vi "Speed Control.vi"(6 "Multiple":dbl, 8 "Down":bool, 9 "Up":bool, 10 "Left Joystick":dbl, 11 "Right Joystick":dbl) -> (0 "Speed":dbl, 2 "Left Motor":dbl, 3 "Right Output":dbl)   [LabVIEW 2016]
doc: "This VI was created to demonstrate common functions used in Labview. It incriments/decrements a value based on the press of Up/Down by a value of multiple. The zero terminal sets the value to zero. The motor input in is multiplied by this value (-1<x<1) to control the maximum speed."
panel:
  in  "Zero":bool
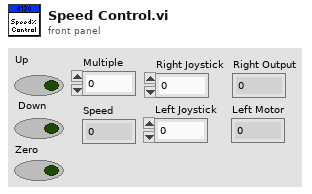
[diagram p1: front panel]
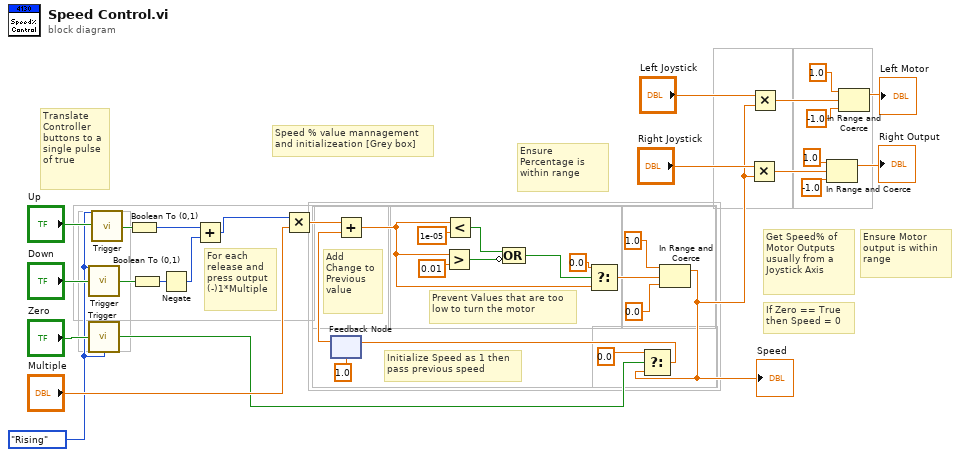
[diagram p0: block diagram]
diagram:
  w1 = enum16{"Falling", "Rising", "Both"}."Rising" ("Enum")
  # "Speed % value mannagement and initializeation [Grey box]"
  # "Get Speed% of Motor Outputs usually from a Joystick Axis"
  # "Ensure Motor output is within range"
  # "Initialize Speed as 1 then pass previous speed"
  # "If Zero == True then Speed = 0"
  # "Ensure Percentage is within range"
  # "Prevent Values that are too low to turn the motor"
  # "For each release and press output (-)1*Multiple"
  # "Translate Controller buttons to a single pulse of true"
  # "Add Change to Previous value"
  n1 = call "Trigger.vi"("Enum"=w1, "Button"="Down") -> ("Trigger"=w27:bool)  [unwired: 13 in]
  n2 = call "Trigger.vi"("Enum"=w1, "Button"="Zero") -> ("Trigger"=w21:bool)  [unwired: 13 in]
  n3 = call "Trigger.vi"("Enum"=w1, "Button"="Up") -> ("Trigger"=w28:bool)  [unwired: 13 in]
  n4 = Boolean To (0,1)(Boolean=w28) -> (0, 1=w33:i16)
  n5 = Boolean To (0,1)(Boolean=w27) -> (0, 1=w2:i16)
  n6 = Negate(x=w2) -> (-x=w3:i16)
  n7 = Add(x=w33, y=w3) -> (x+y=w32:i16)
  n8 = Multiply(x=w32, y="Multiple") -> (x*y=w26:dbl)
  n9 = feedback #1(1.0 ("upper limit")) -> (w31:dbl)
  n10 = Add(x=w26, y=w31) -> (x+y=w7:dbl)
  n11 = Greater?(x=w7, y=0.01) -> (0:w9:bool)
  n12 = Less?(x=w7, y=1e-05) -> (x < y?=w8:bool)
  n13 = Compound Arithmetic op=OR(w8, invert w9) -> (w5:bool)
  n14 = Select(t=0.0, s=w5, f=w7) -> (s? t:f=w4:dbl)
  n15 = In Range and Coerce(upper limit=1.0, x=w4, lower limit=0.0) -> (coerced(x)=w14:dbl)  [unwired: 1 out]
  "Speed" <- w14
  n16 = Select(t=0.0, s=w21, f=w14) -> (s? t:f=w23:dbl)
  n17 = feedback-in #1(w23) -> ()
  n18 = Multiply(x="Right Joystick", y=w14) -> (x*y=w18:dbl)
  n19 = Multiply(x="Left Joystick", y=w14) -> (x*y=w35:dbl)
  n20 = In Range and Coerce(upper limit=1.0, x=w18, lower limit=-1.0) -> (coerced(x)=→"Right Output":dbl)  [unwired: 1 out]
  n21 = In Range and Coerce(upper limit=1.0, x=w35, lower limit=-1.0) -> (coerced(x)=→"Left Motor":dbl)  [unwired: 1 out]
